vi "FPGA_Read.vi"(7 "Offset":u32, 8 "Error_In":errorcluster, 11 "VISA_Rsrc_In":refnum<visa-resource-name>) -> (0 "Error_Out":errorcluster, 2 "Value":u32 format="%x", 3 "VISA_Rsrc_Out":refnum<visa-resource-name>)   [LabVIEW 2018]
uses:
  <vilib>/Instr/_visa.llb/VISA Register Access Address Space.ctl
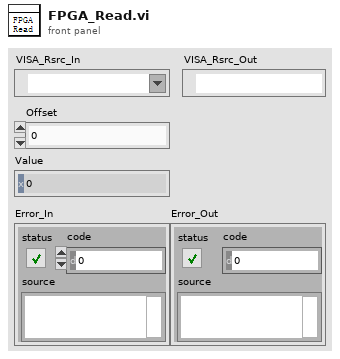
[diagram p1: front panel]
types:
  T1 = typedef "VISA Register Access Address Space.ctl" = u16
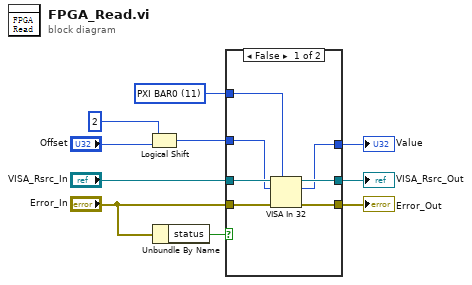
[diagram p0: block diagram]
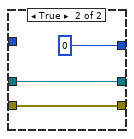
[diagram p2: hidden frame]
diagram:
  w7 = T1 11 items=["VXI/VME A16"=1, "VXI/VME A24"=2, "VXI/VME A32"=3, "VXI/VME A64"=4, "PXI Memory Allocations"=9, "PXI Configuration"=10, "PXI BAR0"=11, "PXI BAR1"=12, "PXI BAR2"=13, "PXI BAR3"=14, "PXI BAR4"=15, "PXI BAR5"=16] ("Address Space")
  n1 = Logical Shift(y=i16 2, x="Offset") -> (x << y=w3:u32)
  n2 = Unbundle By Name("Error_In") -> ("status"=w2:bool)
  n3 = case shown="False" w2 {
    tunnel: "VISA_Rsrc_In" -> [w17 w19]
    tunnel: [w16 w19] -> w9
    tunnel: "Error_In" -> [w15 w18]
    tunnel: [w14 w18] -> w8
    tunnel: w7 -> [w13 _]
    tunnel: [w12 u32 0 ("value")] -> w6
    tunnel: w3 -> [w11 _]
    frame False {
      n4 = VISA In 32(7:w13, 8:w15, 10:w11, 11:w17) -> (0:w14:errorcluster, 2:w12:u32, 3:w16:refnum<visa-resource-name>)
    }
    frame True {
    }
  }
  "VISA_Rsrc_Out" <- w9
  "Error_Out" <- w8
  "Value" <- w6
